vi "GenCVT1Tags.vi"(11 "Number of Tags in":i32=1000) -> (1 "Names":string[](array[string]), 2 "Tags":T1[](array[typedef]), 3 "Number of Tags out":i32)   [LabVIEW 2013, in "UnitTests.lvlib"]
uses:
  UnitTests.lvlib
  <vilib>/NI/Current Value Table/Compatibility/_SubVIs/TypeDefs/cvt_Tag Configuration.ctl
  <vilib>/NI/Current Value Table/Compatibility/_SubVIs/TypeDefs/cvt_Data Types.ctl
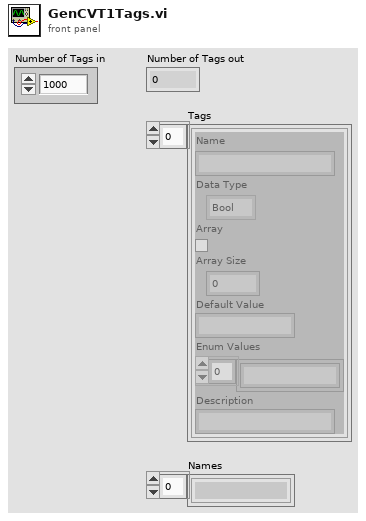
[diagram p1: front panel]
types:
  T1 = typedef "cvt_Tag Configuration.ctl" = cluster{"Name":string, "Data Type":T2, "Array":bool, "Size":u32, "Default":string, "Enum":string[], "Description":string}
  T2 = typedef "cvt_Data Types.ctl" = enum16{"Bool", "U8", "I32", "Double", "String", "Enum"}
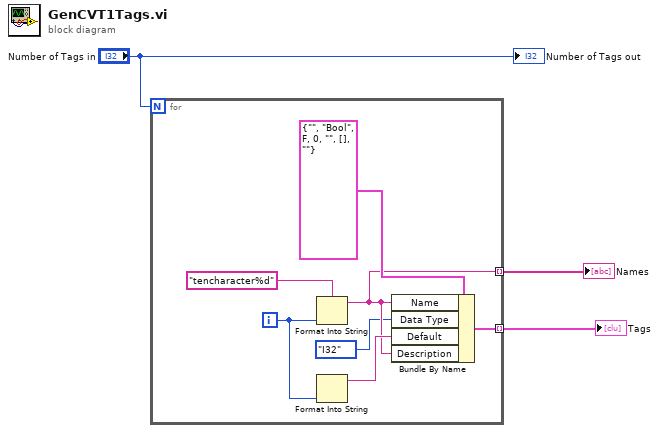
[diagram p0: block diagram]
diagram:
  n1 = for {
    N: "Number of Tags in" -> [_]
    tunnel: [w9] -> w2 mode=indexing
    tunnel: [w5] -> w1 mode=indexing
    i -> [w7]
    n2 = Format Into String(format string="tencharacter%d", w7) -> (resulting string=w5:string)  [unwired: 2 in, 1 out]
    n3 = Format Into String(w7) -> (resulting string=w6:string)  [unwired: 3 in, 1 out]
    n4 = Bundle By Name(cluster=T1 {"Name"="", "Data Type"=enum."Bool", "Array"=FALSE, "Size"=0, "Default"="", "Enum"=[], "Description"=""} ("Tag"), "Name"=w5, "Data Type"=cvt_Data_Types."I32", "Default"=w6, "Description"=w5) -> (w9:T1)
  }
  "Tags" <- w2
  "Names" <- w1
  "Number of Tags out" <- "Number of Tags in"
